vi "Bus_Monitor_API StreamBus Read.vi"(8 "error in":errorcluster, 11 "Call ID in":T7) -> (0 "error out":errorcluster, 1 "Success":bool, 2 "Response Data":T1, 3 "Call ID":T7)   [LabVIEW 2025, in "bus_monitor_client.lvlib"]
uses:
  bus_monitor_client.lvlib
  <vilib>/gRPC/LabVIEW gRPC Library/Shared/grpcId.ctl
  RPC Messages/ni_bus_monitor_api_StreamBusReply.ctl
  RPC Messages/ni_bus_monitor_api_CanCommState.ctl
  RPC Messages/ni_bus_monitor_api_CommState.ctl
  RPC Messages/ni_bus_monitor_api_LastCommError.ctl
  RPC Messages/ni_bus_monitor_api_Frame.ctl
  RPC Messages/ni_bus_monitor_api_ErrorInfo.ctl
  RPC Messages/ni_bus_monitor_api_StreamBusReply_Flat.ctl
  RPC Messages/ni_bus_monitor_api_CanCommState_Flat.ctl
  RPC Messages/ni_bus_monitor_api_Frame_Flat.ctl
  RPC Messages/ni_bus_monitor_api_ErrorInfo_Flat.ctl
  aea5dbbb-03a2-479b-ad95-94da4ee1cea9.vi
  <vilib>/gRPC/LabVIEW gRPC Library/Shared/TranslateGrpcError.vi
  <vilib>/gRPC/LabVIEW gRPC Library/Shared/Wait On Occurrence.vi
  RPC Messages/FlatToRichni_bus_monitor_api_CanCommState.vi
  RPC Messages/FlatToRichni_bus_monitor_api_Frame.vi
  RPC Messages/FlatToRichni_bus_monitor_api_ErrorInfo.vi
  <vilib>/gRPC/LabVIEW gRPC Library/Shared/Is Feature Enabled.vi
  <vilib>/gRPC/LabVIEW gRPC Library/Server API/Server/Get Server DLL Path.vi
  <vilib>/Utility/error.llb/Error Cluster From Error Code.vi
  <vilib>/gRPC/LabVIEW gRPC Library/grpc-lvsupport-release.lvlib
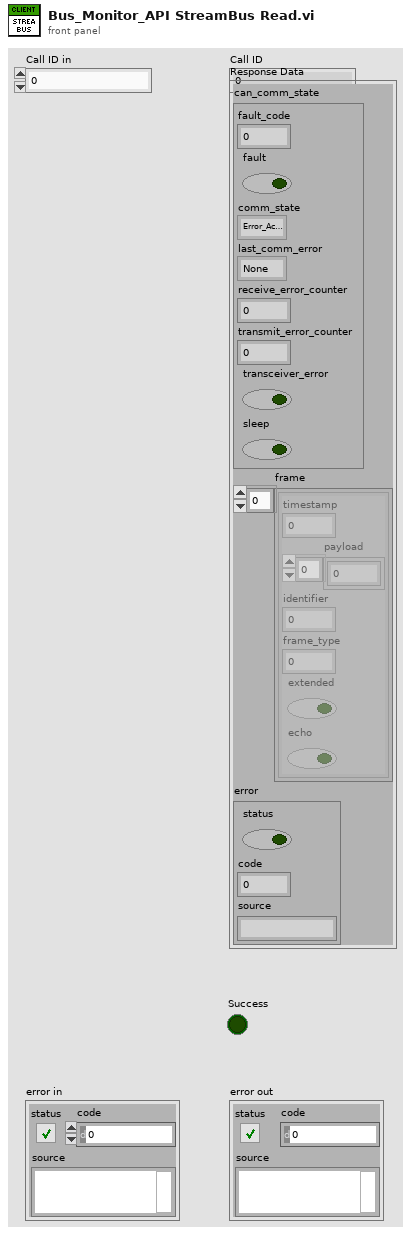
[diagram p1: front panel]
types:
  T1 = typedef "bus_monitor_client.lvlib/ni_bus_monitor_api_StreamBusReply.ctl" = cluster{"can_comm_state":T2, "frame":T5[], "error":T6}
  T2 = typedef "bus_monitor_client.lvlib/ni_bus_monitor_api_CanCommState.ctl" = cluster{"fault_code":i32, "fault":bool, "comm_state":T3, "last_comm_error":T4, "receive_error_counter":u32, "transmit_error_counter":u32, "transceiver_error":bool, "sleep":bool}
  T3 = typedef "bus_monitor_client.lvlib/ni_bus_monitor_api_CommState.ctl" = enum32{"Error_Active", "Error_Passive", "Bus_Off", "Init"}
  T4 = typedef "bus_monitor_client.lvlib/ni_bus_monitor_api_LastCommError.ctl" = enum32{"None", "Stuff", "Form", "ACK", "Bit1", "Bit0", "CRC"}
  T5 = typedef "bus_monitor_client.lvlib/ni_bus_monitor_api_Frame.ctl" = cluster{"timestamp":dbl, "payload":u8[], "identifier":u32, "frame_type":u32, "extended":bool, "echo":bool}
  T6 = typedef "bus_monitor_client.lvlib/ni_bus_monitor_api_ErrorInfo.ctl" = errorcluster
  T7 = typedef "grpc-lvsupport-release.lvlib/grpcId.ctl" = u64
  T8 = typedef "bus_monitor_client.lvlib/ni_bus_monitor_api_StreamBusReply_Flat.ctl" = cluster{"can_comm_state":T9, "frame":T10[], "error":T11}
  T9 = typedef "bus_monitor_client.lvlib/ni_bus_monitor_api_CanCommState_Flat.ctl" = cluster{"fault_code":i32, "fault":bool, "comm_state":T3, "last_comm_error":T4, "receive_error_counter":u32, "transmit_error_counter":u32, "transceiver_error":bool, "sleep":bool}
  T10 = typedef "bus_monitor_client.lvlib/ni_bus_monitor_api_Frame_Flat.ctl" = cluster{"timestamp":dbl, "payload":u8[], "identifier":u32, "frame_type":u32, "extended":bool, "echo":bool}
  T11 = typedef "bus_monitor_client.lvlib/ni_bus_monitor_api_ErrorInfo_Flat.ctl" = errorcluster
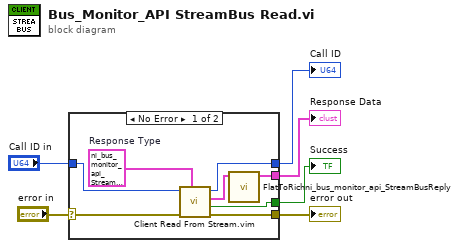
[diagram p0: block diagram]
diagram:
  n1 = case shown="No Error" "error in" {
    selector: "error in" -> [w14 w15]
    tunnel: [w13 w15] -> w5
    tunnel: "Call ID in" -> [w12 w16]
    tunnel: [w10 w16] -> w3
    tunnel: [w7 _] -> w2
    tunnel: [w11 _] -> w1
    frame No Error {
      w9 = T8 {"can_comm_state"={"fault_code"=0, "fault"=FALSE, "comm_state"=enum."Error_Active", "last_comm_error"=enum."None", "receive_error_counter"=0, "transmit_error_counter"=0, "transceiver_error"=FALSE, "sleep"=FALSE}, "frame"=[], "error"={"status"=FALSE, "code"=0, "source"=""}}  # Response Type
      n2 = call "Client Read From Stream.vim"("Response Type"=w9, "error in"=w14, "Call ID in"=w12) -> ("error out"=w13:errorcluster, "Success"=w11:bool, "Response Data"=w8:T8, "Call ID out"=w10:u64)  [unwired: 5 in]
      n3 = call "FlatToRichni_bus_monitor_api_StreamBusReply.vi"("InputCluster"=w8) -> ("OutputCluster"=w7:T1)  [unwired: 10 in]
    }
    frame Error {
    }
  }
  "error out" <- w5
  "Call ID" <- w3
  "Response Data" <- w2
  "Success" <- w1
